vi "Browse FOM RTM.vi"(8 "error in":errorcluster, 11 "Node Ptr":u64 format="%.0x") -> (0 "error out":errorcluster)   [LabVIEW 2019, in "HLA Custom Device System Explorer.lvlib"]
uses:
  HLA Custom Device System Explorer.lvlib
  FOM/_typedefs/object_instance_json_type.ctl
  FOM/_typedefs/interaction_json_type.ctl
  <vilib>/Utility/SystemLogging/NI_SystemLogging.lvlib
panel:
  out "Interactions":T1[](array[typedef])
  out "Objects":T2[](array[typedef])
  in  "load":bool
  in  "FOM File Path":path
  in  "cancel":bool
  in  "ok":bool
  in  "Tag":string
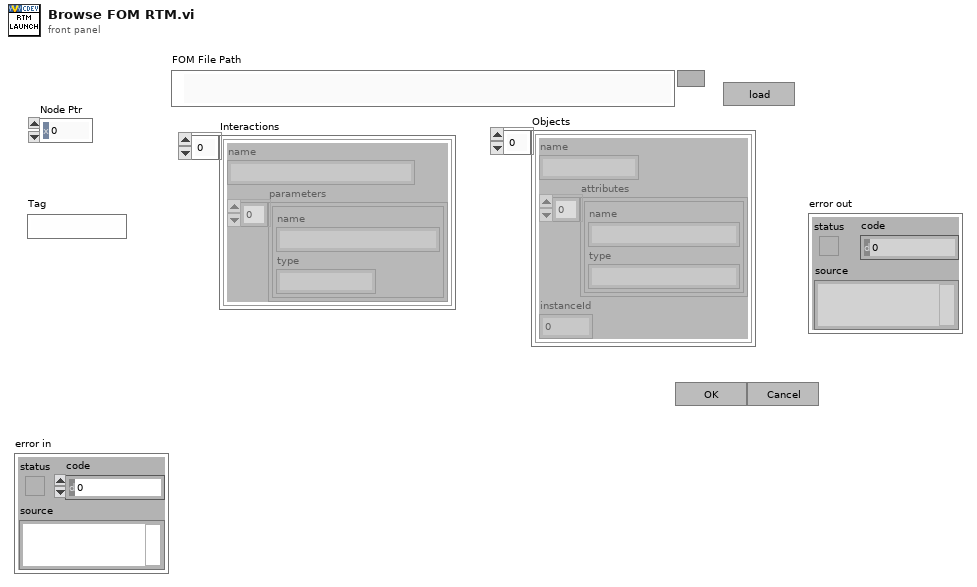
[diagram p1: front panel]
types:
  T1 = typedef "HLA Custom Device System Explorer.lvlib/interaction_json_type.ctl" = cluster{"name":string, "parameters":cluster{"name":string, "type":string}[]}
  T2 = typedef "HLA Custom Device System Explorer.lvlib/object_instance_json_type.ctl" = cluster{"name":string, "attributes":cluster{"name":string, "type":string}[], "instanceId":i32}
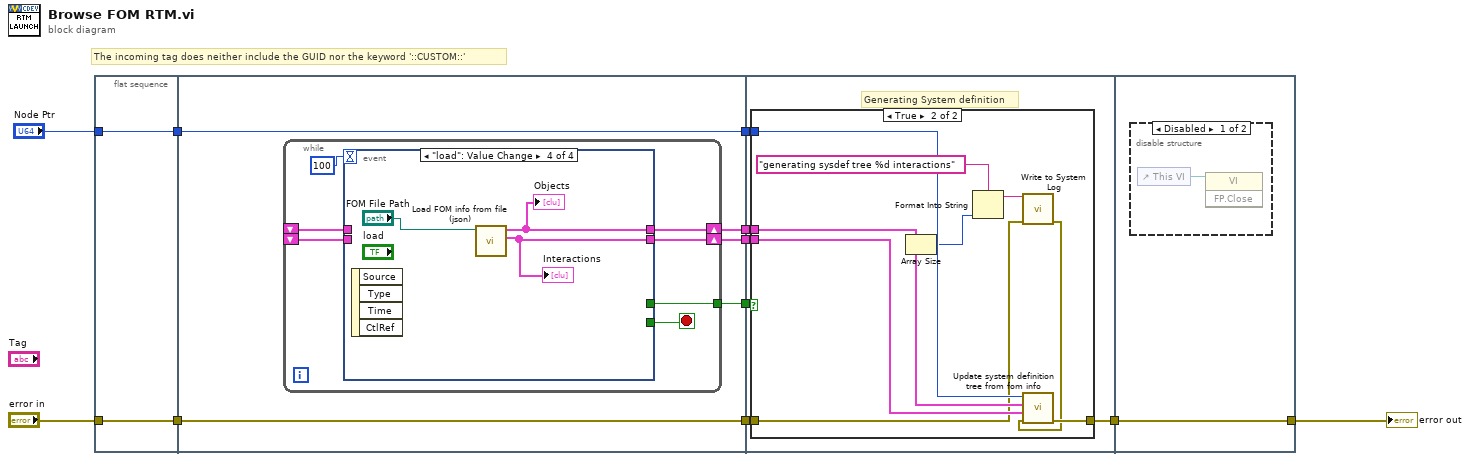
[diagram p0: block diagram]
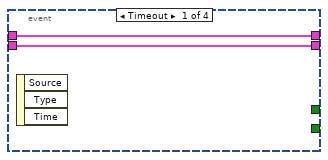
[diagram p2: hidden frame]
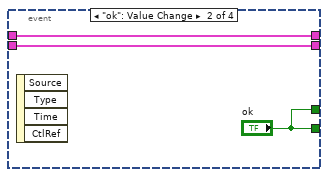
[diagram p3: hidden frame]
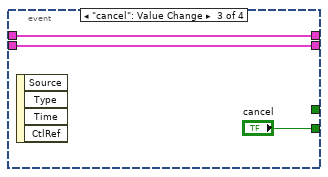
[diagram p4: hidden frame]
diagram:
  # "The incoming tag does neither include the GUID nor the keyword '::CUSTOM::'"
  n1 = flat-sequence {
    tunnel: [w13] -> w9
    tunnel: "Node Ptr" -> [w13]
    tunnel: [w12] -> w6
    tunnel: "error in" -> [w12]
    tunnel: [w18] -> w11
    tunnel: [w17] -> w10
    tunnel: w9 -> [w17]
    tunnel: [w16] -> w7
    tunnel: w6 -> [w16]
    tunnel: [w15] -> w2
    tunnel: [w14] -> w1
    tunnel: w11 -> [w42]
    tunnel: w10 -> [w41]
    tunnel: w7 -> [w40]
    tunnel: [w39] -> w3
    tunnel: w2 -> [w38]
    tunnel: w1 -> [w37]
    tunnel: [w53] -> w4
    tunnel: w3 -> [w53]
    frame #0 {
    }
    frame #1 {
      n2 = while {
        tunnel: [w23] -> w18
        shift-right: [w22] -> w15
        shift-left: _ -> [w20]
        shift-right: [w21] -> w14
        shift-left: _ -> [w19]
        stop <- w25 stop-if-true
        n3 = event shown="[3] \"load\": Value Change" {
          selector: _ -> [_ _ _ _]
          dyn-events: _ -> [_ _ _ _]
          timeout: 100 -> [_ _ _ _]
          tunnel: [_ "ok" "cancel" _] -> w25
          tunnel: [_ "ok" _ _] -> w23
          tunnel: [w27 w29 w32 w35] -> w22
          tunnel: [w26 w28 w31 w34] -> w21
          tunnel: w20 -> [w27 w29 w32 _]
          tunnel: w19 -> [w26 w28 w31 _]
          event Timeout {
            n4 = event-data() -> ()  [unwired: 1 in, 3 out]
          }
          event "ok": Value Change {
            n5 = event-data() -> ()  [unwired: 1 in, 4 out]
          }
          event "cancel": Value Change {
            n6 = event-data() -> ()  [unwired: 1 in, 4 out]
          }
          event "load": Value Change {
            n7 = event-data() -> ()  [unwired: 1 in, 4 out]
            n8 = call "Load FOM info from file (json).vi"("fom export"="FOM File Path") -> ("Interactions"=w34:T1[], "Objects"=w35:T2[])  [unwired: 8 in, 1 out]
            "Objects" <- w35
            "Interactions" <- w34
          }
        }
      }
    }
    frame #2 {
      # "Generating System definition"
      n9 = case shown="True" w42 {
        tunnel: w41 -> [_ w51]
        tunnel: w40 -> [w43 w45]
        tunnel: [w43 w52] -> w39
        tunnel: w38 -> [_ w49]
        tunnel: w37 -> [_ w50]
        frame False {
        }
        frame True {
          n10 = Array Size(array=w49) -> (size(s)=w48:i32)
          n11 = Format Into String(format string="generating sysdef tree %d interactions", w48) -> (resulting string=w47:string)  [unwired: 2 in, 1 out]
          n12 = call <vilib>:"Write to System Log.vi"("error in (no error)"=w45, "message"=w47) -> ("error out"=w44:errorcluster)  [unwired: 9 in]
          n13 = call "Update system definition tree from fom info.vi"("error in"=w44, "Interactions"=w50, "Objects"=w49, "Item Ref in"=w51) -> ("error out"=w52:errorcluster)  [unwired: 6 in, 1 out]
        }
      }
    }
    frame #3 {
      n14 = disable-structure shown="Disabled" {
        frame Disabled {
          n15 = control-ref of="This VI"() -> (w54:refnum<vi>)
          n16 = invoke class="VI" method="FP.Close"(reference=w54) -> ()  [unwired: 2 in, 3 out]
        }
        frame Enabled {
        }
      }
    }
  }
  "error out" <- w4
